vi "oscilloscopio_vero.vi"() -> ()   [LabVIEW 2018]
uses:
  <vilib>/Utility/error.llb/DialogType.ctl
panel:
  out "frequenza \n[Hz]":dbl
  in  "isteresi":dbl=0.10000000000000003 min=0.0 max=2.0 step=0.1
  in  "livello":dbl min=0.0 step=0.5
  in  "% trigger":dbl(slide) min=0.0 max=100.0 step=10.0 scale=0.0..100.0
  in  "?":bool
  out "Rms Ch 2":dbl=1.0694672854571177 format="%.3f"
  out "Rms Ch 1":dbl=1.768275149331526 format="%.3f"
  out "S P.Apparente[VA]":dbl=1.8911124238968666 format="%.3f"
  out "Q P.Reattiva[VAr]":dbl=1.3129600353014463 format="%.3f"
  out "P attiva[W]":dbl=-1.361044505340772 format="%.3f"
  in  "?":bool=TRUE
  in  "s/Div":dbl(ring)=0.002 items=["100ms"=0.1, "50ms"=0.05, "20ms"=0.02, "10ms"=0.01, "5ms"=0.005, "2ms"=0.002, "1ms"=0.001]
  in  "Volt/Div Ch 2":dbl(ring)=1.0 items=["10V"=10.0, "5V"=5.0, "2V"=2.0, "1V"=1.0, "500mV"=0.5, "200mV"=0.2, "100mV"=0.1, "50mV"=0.05, "20mV"=0.02, "10mV"=0.01]
  in  "Volt/Div Ch 1":dbl(ring)=1.0 items=["10V"=10.0, "5V"=5.0, "2V"=2.0, "1V"=1.0, "500mV"=0.5, "200mV"=0.2, "100mV"=0.1, "50mV"=0.05, "20mV"=0.02, "10mV"=0.01]
  in  "?":bool
  out "?":waveform(dbl)[](graph)=[{"t0"=timestamp(3719217833.313895 s since 1904-01-01), "dt"=4.999999999999959e-06, "Y"=array[4000 elements], "attributes"=variant("NI_ChannelName"=variant(string "PXIe_NI6341/ai1"), "NI_UnitDescription"=variant(string "Volts"))}, {"t0"=timestamp(3719217833.313895 s since 1904-01-01), "dt"=4.999999999999959e-06, "Y"=array[4000 elements], "attributes"=variant("NI_ChannelName"=variant(string "PXIe_NI6341/ai1"), "NI_UnitDescription"=variant(string "Volts"))}]
  out "ultimo trigger":i32=2840
  out "1 Trigger":i32=340
  out "valore di picco":dbl=2.4867874882116237
  out "valore di picco":dbl=2.4867874882116237
  in  "N":dbl=1000.0 min=2.0 step=100.0
  out "2 segnale":dbl[](array[numeric])
  out "1 segnale":dbl[](array[numeric])
  # "TRIGGER"
  # "SCELTA"
  # "HORIZONTAL"
  # "MODALITY"
  # "VERTICAL"
  # "salita"
  # "discesa"
  # "Ch 1"
  # "Ch 2"
  # "Ch 1"
  # "Ch 2"
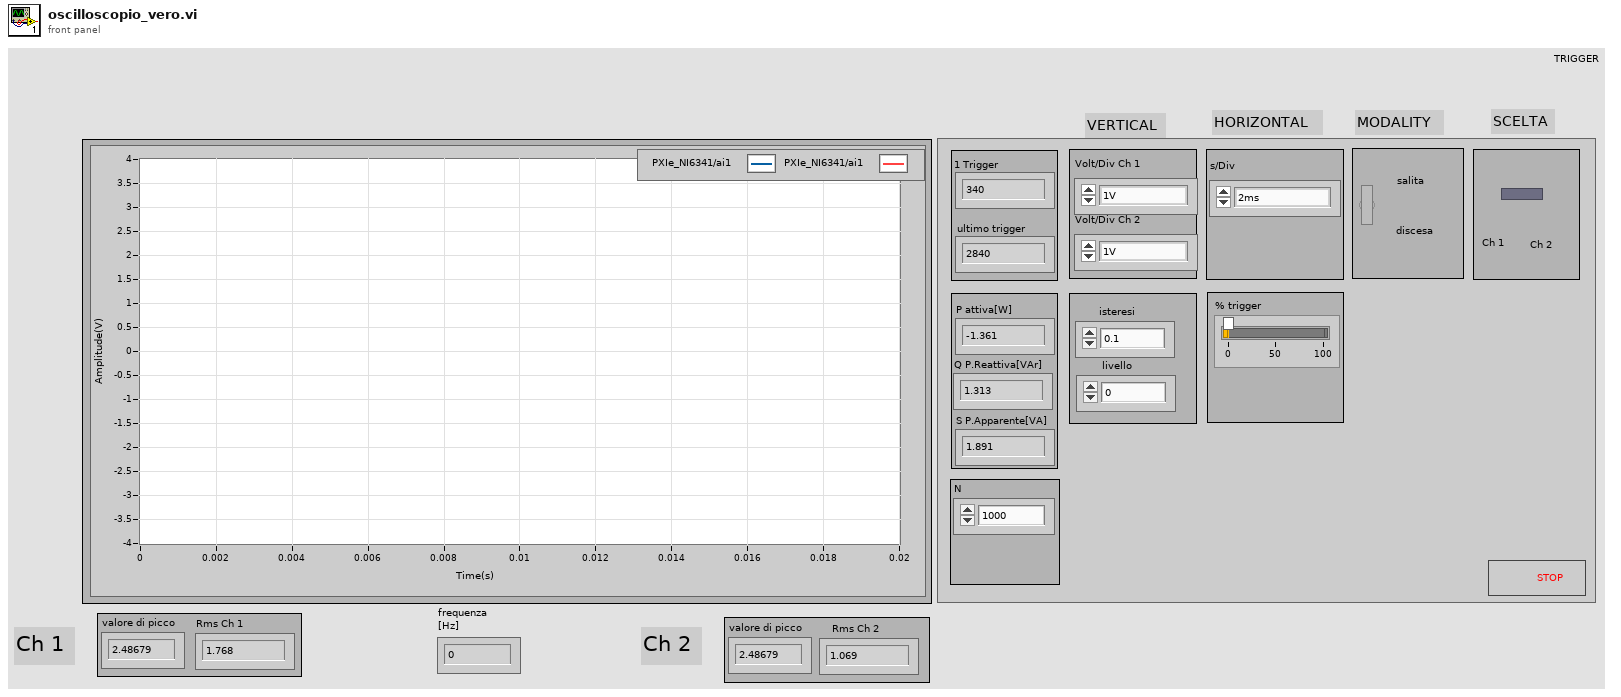
[diagram p1: front panel]
types:
  T1 = typedef "DialogType.ctl" = u16
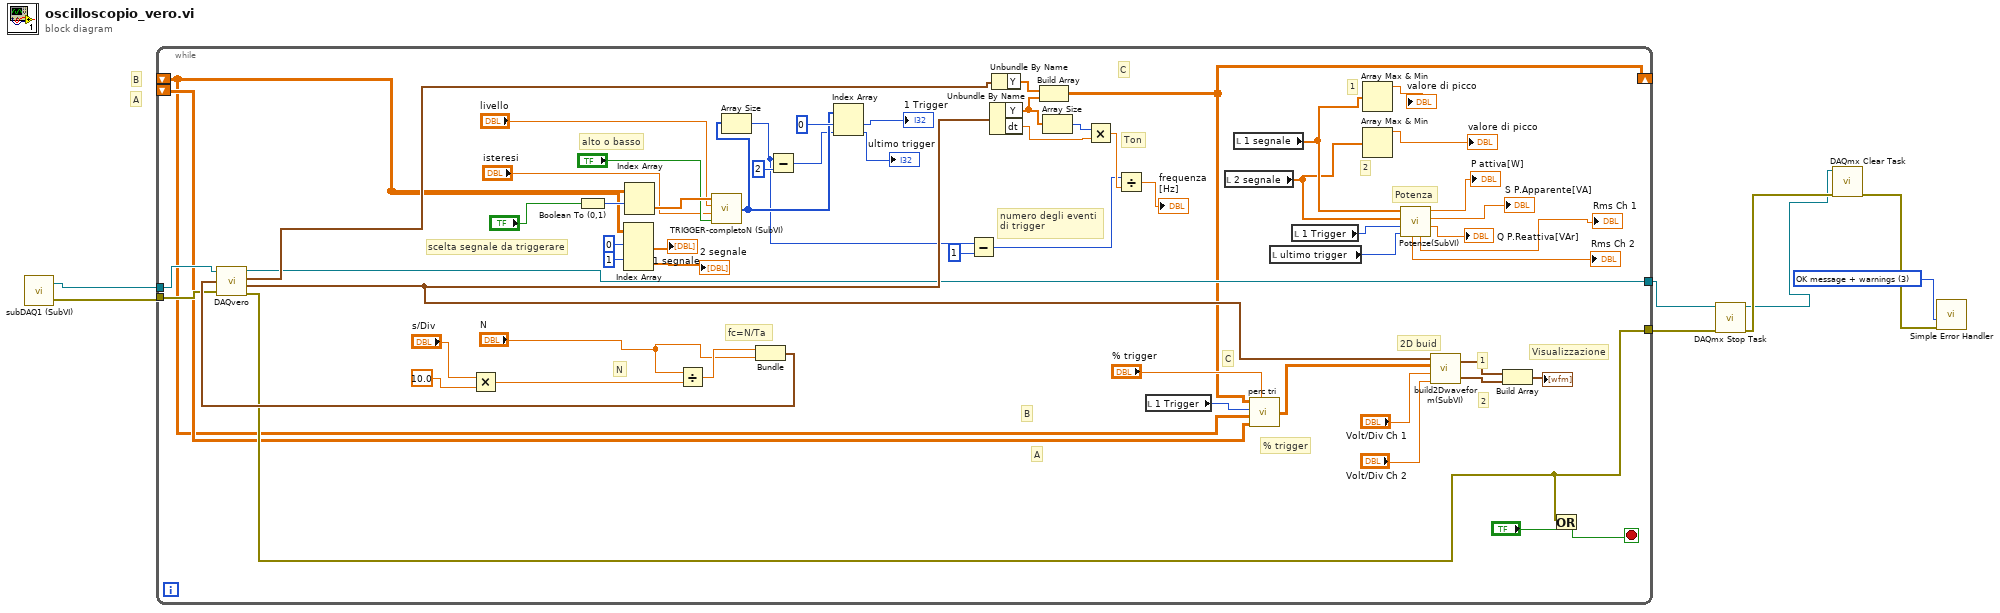
[diagram p0: block diagram]
diagram:
  w5 = T1 3 items=["no dialog", "OK message", "continue or stop message", "OK message + warnings", "continue/stop + warnings"] ("type of dialog (OK msg:1)")
  # "A"
  # "B"
  n1 = call "subDAQ1 (SubVI).vi"() -> ("error out"=w1:errorcluster, "Refnum out"=w2:refnum<k21>)  [unwired: 3 in]
  n2 = while {
    shift-right: [w12] -> _
    shift-left: _ -> [w9]
    shift-left: _ -> [w10]
    tunnel: w2 -> [w57]
    tunnel: [w54] -> w4
    tunnel: w1 -> [w53]
    tunnel: [w49] -> w3
    stop <- w50 stop-if-true
    # "fc=N/Ta"
    # "numero degli eventi\ndi trigger"
    # "Ton"
    # "alto o basso"
    # "scelta segnale da triggerare"
    # "1"
    # "2"
    # "N"
    # "Visualizzazione"
    # "2"
    # "1"
    # "Potenza"
    # "2D buid"
    # "% trigger"
    # "B"
    # "A"
    # "C"
    # "C"
    n3 = Multiply(x="s/Div", y=10.0) -> (x*y=w68:dbl)
    n4 = Boolean To (0,1)(Boolean="?") -> (0, 1=w66:i16)
    n5 = Index Array(array=w9, index (row) #1=0 ("index (row)"), index (row) #2=1 ("index (row)")) -> (element #1=→"1 segnale":dbl[], element #2=→"2 segnale":dbl[])  [unwired: 2 in]
    n6 = Index Array(array=w9, index (row)=w66) -> (element=w65:dbl[])  [unwired: 1 in]
    n7 = Divide(x="N", y=w68) -> (x/y=w67:dbl)
    n8 = call "TRIGGER-completoN (SubVI).vi"("Modalità"="?", "isteresi"="isteresi", "livello"="livello", "Segnale B"=w65) -> ("eventi di trigger"=w30:i32[])
    n9 = Array Size(array=w30) -> (size(s)=w18:i32)
    n10 = Bundle(w67, "N"="N") -> (w58:cluster{dbl, "N":dbl})  [unwired: 1 in]
    n11 = call "DAQvero.vi"("task/channels in"=w57, "sampling info"=w58, "error in"=w53) -> ("task out"=w54:refnum<k21>, "1 segnale"=w56:waveform(dbl), "2 segnale"=w55:waveform(dbl), "error out"=w49:errorcluster)
    n12 = Subtract(x=w18, y=2) -> (x-y=w29:i32)
    n13 = Index Array(array=w30, index #1=0 ("index"), index #2=w29) -> (element #1=→"1 Trigger":i32, element #2=→"ultimo trigger":i32)
    n14 = Subtract(x=w18, y=1) -> (x-y=w16:i32)
    n15 = Unbundle By Name(w55) -> ("Y"=w21:dbl[], "dt"=w20:dbl)
    n16 = Unbundle By Name(w56) -> ("Y"=w59:dbl[])
    n17 = Build Array(w59, w21) -> (w12:dbl[][])
    n18 = Array Size(array=w21) -> (size(s)=w22:i32)
    n19 = Multiply(x=w22, y=w20) -> (x*y=w19:dbl)
    n20 = Divide(x=w16, y=w19) -> (x/y=→"frequenza \n[Hz]":dbl)
    n21 = local read "1 Trigger"() -> (w11:i32)
    n22 = local read "2 segnale"() -> (w25:dbl[])
    n23 = local read "1 segnale"() -> (w26:dbl[])
    n24 = call "perc tri.vi"("C"=w12, "trigger"=w11, "B"=w9, "A"=w10, "%"="% trigger") -> ("Array"=w14:dbl[][])
    n25 = local read "ultimo trigger"() -> (w24:i32)
    n26 = local read "1 Trigger"() -> (w23:i32)
    n27 = Array Max & Min(array=w26) -> (max value=→"valore di picco":dbl)  [unwired: 3 out]
    n28 = Array Max & Min(array=w25) -> (max value=→"valore di picco":dbl)  [unwired: 3 out]
    n29 = call "Potenze(SubVI).vi"("ultimo trigger"=w24, "1 trigger"=w23, "2"=w25, "1"=w26) -> ("Q P.Reattiva"=→"Q P.Reattiva[VAr]":dbl, "S P.Apparente"=→"S P.Apparente[VA]":dbl, "P attiva"=→"P attiva[W]":dbl, "Rms Ch 1"=→"Rms Ch 1":dbl, "Rms Ch 2"=→"Rms Ch 2":dbl)  [unwired: 3 in]
    n30 = call "build2Dwaveform(SubVI).vi"("Volt/Div Ch 2"="Volt/Div Ch 2", "Volt/Div Ch 1"="Volt/Div Ch 1", "Array"=w14, "waveform"=w55) -> ("secondo segnale"=w61:waveform(dbl), "primo segnale"=w62:waveform(dbl))
    n31 = Build Array(w62, w61) -> (→"?":waveform(dbl)[])
    n32 = Or(x=w49, y="?") -> (x .or. y?=w50:bool)
  }
  n33 = call <vilib>:"DAQmx Stop Task.vi"("task/channels in"=w4, "error in"=w3) -> ("task out"=w6:refnum<k21>, "error out"=w7:errorcluster)  [unwired: 12 in]
  n34 = call <vilib>:"DAQmx Clear Task.vi"("task in"=w6, "error in"=w7) -> ("error out"=w8:errorcluster)  [unwired: 13 in]
  n35 = call <vilib>:"Simple Error Handler.vi"("type of dialog (OK msg:1)"=w5, "error in (no error)"=w8) -> ()  [unwired: 3 in, 5 out]
